vi "Read database.vi"(8 "error in (no error)":errorcluster caption="错误输入（无错误）", 9 "condition":string="where 时间 between #2020/03/27 14:26:18 # and #2020/04/26 14:26:18# order by 时间 desc", 10 "组合框":string(combo)="CODMn", 11 "database":string="database1.mdb") -> (0 "error out":errorcluster caption="错误输出", 2 "column information":T2(array[cluster]), 3 "表格":string[][](table))   [LabVIEW 2016]
uses:
  <vilib>/addons/database/Auxilliary.llb/DB Tools DataTypes.ctl
  <vilib>/Utility/sysdir.llb/System Directory Type.ctl
  <vilib>/addons/database/Connection.llb/DB Tools Open Connec (String).vi
  <vilib>/addons/database/_DB Variant To Data/Database Variant To Data.xnode
  <vilib>/addons/database/NI_Database_API.lvlib
panel:
  in  "精度(6)":i16=2
  in  "显示项":string[](array[string])
  out "columns":string[](array[string])
  out "data":variant[][](array[variant])
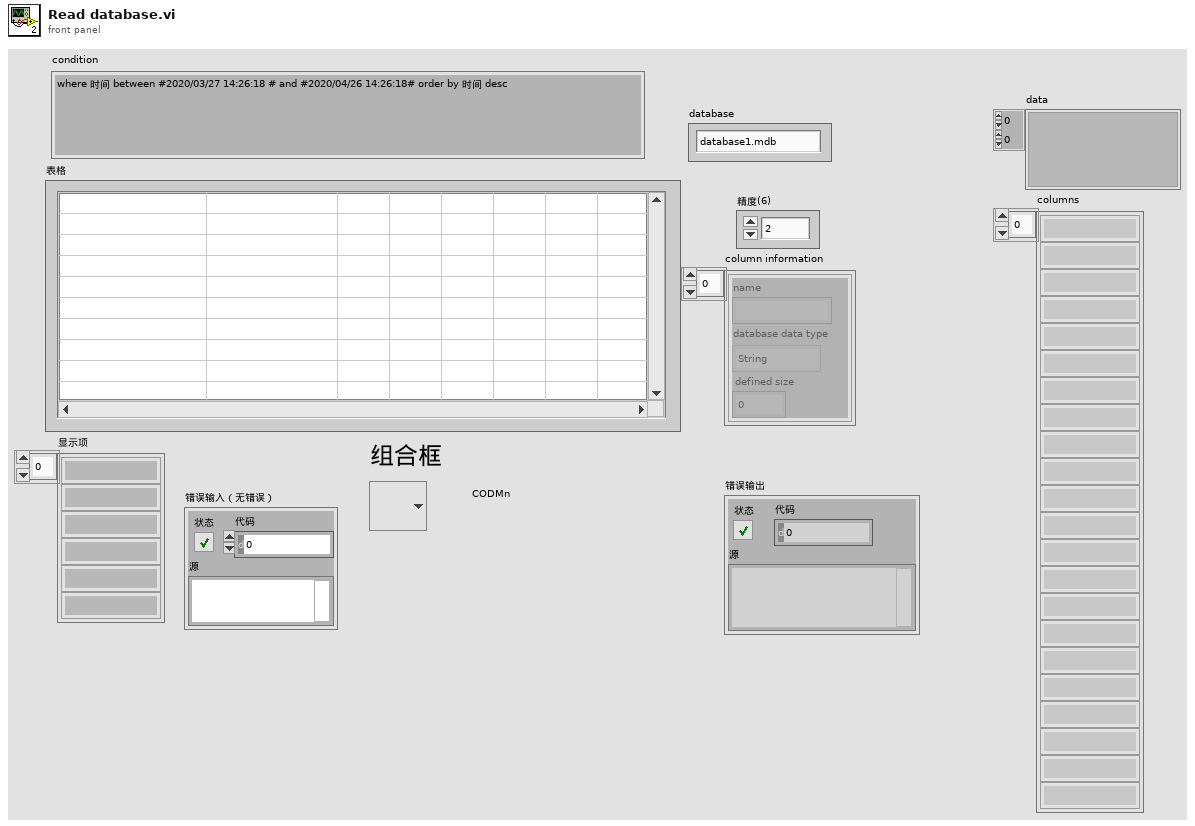
[diagram p1: front panel]
types:
  T1 = typedef "NI_Database_API.lvlib/DB Tools DataTypes.ctl" = enum16{"String", "Long (I32)", "Single (SGL)", "Double (DBL)", "Date/Time", "Binary"}
  T2 = cluster{"name":string, "database data type":T1, "defined size":i32}[]
  T3 = typedef "System Directory Type.ctl" = i32
  T4 = typedef "NI_Database_API.lvlib/Conn ObjectReference.ctl" = refnum<k1>
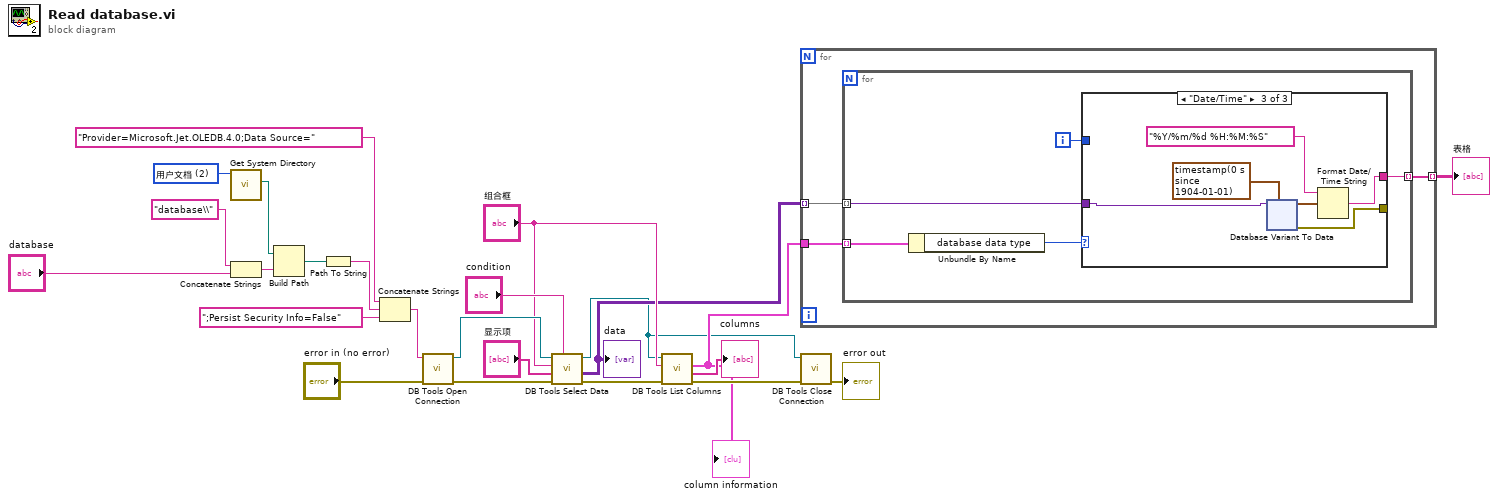
[diagram p0: block diagram]
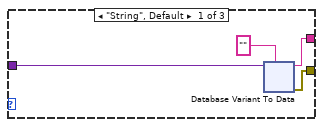
[diagram p2: hidden frame]
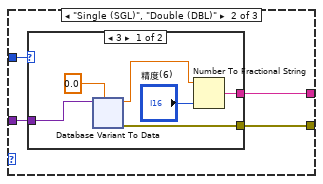
[diagram p3: hidden frame]
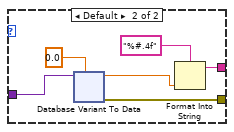
[diagram p4: hidden frame]
diagram:
  w11 = T3 2 items=["用户目录"=0, "用户桌面"=1, "用户文档"=2, "用户应用程序数据"=3, "用户设置"=4, "用户临时目录"=5, "公共文档"=6, "公共应用程序数据"=7, "公共设置"=8, "公共缓存"=13, "系统核心库"=9, "系统安装库"=10, "应用程序文件"=11, "启动盘根目录"=12] ("system directory type")
  n1 = call <vilib>:"Get System Directory.vi"("system directory type"=w11) -> ("system directory"=w10:path)  [unwired: 10 in]
  n2 = Concatenate Strings("database\\" ("名称或相对路径"), "database") -> (w7:string)
  n3 = Build Path(base path=w10, name or relative path=w7) -> (appended path=w12:path)
  n4 = Path To String(path=w12) -> (string=w13:string)
  n5 = Concatenate Strings("Provider=Microsoft.Jet.OLEDB.4.0;Data Source=", w13, ";Persist Security Info=False") -> (w9:string)
  n6 = call-poly <vilib>:"DB Tools Open Connection.vi"("error in (no error)"="error in (no error)", "connection information"=w9) -> ("error out"=w23:errorcluster, "connection reference"=w24:T4)  [unwired: 6 in]
  n7 = call <vilib>:"DB Tools Select Data.vi"("condition"="condition", "error in (no error)"=w23, "columns"="显示项", "table"="组合框", "connection reference"=w24) -> ("error out"=w22:errorcluster, "data"=w4:variant[][], "connection reference out"=w1:T4)  [unwired: 1 in]
  "data" <- w4
  n8 = call <vilib>:"DB Tools List Columns.vi"("error in (no error)"=w22, "table"="组合框", "connection reference"=w1) -> ("error out"=w16:errorcluster, "columns"=→"columns":string[], "column information"=w3:T2)  [unwired: 1 in, 1 out]
  "column information" <- w3
  n9 = for {
    tunnel: w4 -> [w27] mode=indexing
    tunnel: w3 -> [w26]
    tunnel: [w25] -> w2 mode=indexing
    n10 = for {
      tunnel: w27 -> [w31] mode=indexing
      tunnel: w26 -> [w30] mode=indexing
      tunnel: [w28] -> w25 mode=indexing
      i -> [w29]
      n11 = Unbundle By Name(w30) -> ("database data type"=w32:T1)
      n12 = case shown="\"Date/Time\"" w32 {
        tunnel: w31 -> [w36 w72 w154]
        tunnel: [w35 w71 w150] -> w28
        tunnel: w29 -> [_ w70 _]
        tunnel: [w33 w69 w149] -> _
        frame "String", Default {
          n13 = xnode "Database Variant To Data"("database variant"=w36, "type"="") -> ("data"=w35:string, "error out"=w33:errorcluster)  [unwired: 1 in]
        }
        frame "Single (SGL)", "Double (DBL)" {
          n14 = case shown="3" w70 {
            tunnel: w72 -> [w78 w116]
            tunnel: [w76 w114] -> w71
            tunnel: [w73 w111] -> w69
            frame 3 {
              n15 = xnode "Database Variant To Data"("database variant"=w78, "type"=0.0) -> ("data"=w77:dbl, "error out"=w73:errorcluster)  [unwired: 1 in]
              n16 = Number To Fractional String(number=w77, precision (6)="精度(6)") -> (F-format string=w76:string)  [unwired: 2 in]
            }
            frame Default {
              n17 = xnode "Database Variant To Data"("database variant"=w116, "type"=0.0) -> ("data"=w115:dbl, "error out"=w111:errorcluster)  [unwired: 1 in]
              n18 = Format Into String(format string="%#.4f" ("格式字符串"), w115) -> (resulting string=w114:string)  [unwired: 2 in, 1 out]
            }
          }
        }
        frame "Date/Time" {
          n19 = xnode "Database Variant To Data"("database variant"=w154, "type"=timestamp(0 s since 1904-01-01) ("当前时间")) -> ("data"=w153:timestamp, "error out"=w149:errorcluster)  [unwired: 1 in]
          n20 = Format Date/Time String(time format string (%c)="%Y/%m/%d %H:%M:%S" ("时间格式字符串(%c)"), seconds (now)=w153) -> (date/time string=w150:string)  [unwired: 1 in]
        }
      }
    }
  }
  "表格" <- w2
  n21 = call <vilib>:"DB Tools Close Connection.vi"("error in (no error)"=w16, "connection reference"=w1) -> ("error out"=→"error out":errorcluster)  [unwired: 5 in]
